vi "SendMailIfError.vi"(11 "error in (no error)":errorcluster) -> ()   [LabVIEW 2013]
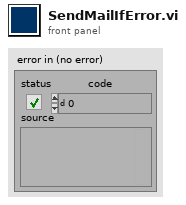
[diagram p1: front panel]
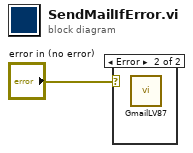
[diagram p0: block diagram]
diagram:
  n1 = case shown="Error" "error in (no error)" {
    frame No Error {
    }
    frame Error {
      n2 = call "GmailLV87.vi"() -> ()  [unwired: 1 in]
    }
  }
